vi "Parse Lights JSON.vi"(8 "error in":errorcluster, 10 "Light JSON":string="{\"1\":{\"name\": \"Hue Lamp\"},\"2\":{\"name\": \"Hue Lamp 1\"},\"3\":{\"name\": \"Hue Lamp 2\"}}") -> (0 "error out":errorcluster, 2 "Light Map":map{i32, T1}(c390))   [LabVIEW 2020, in "LMH-Hue.lvlib"]
uses:
  LMH-Hue.lvlib
  Type Defs/Light Data.ctl
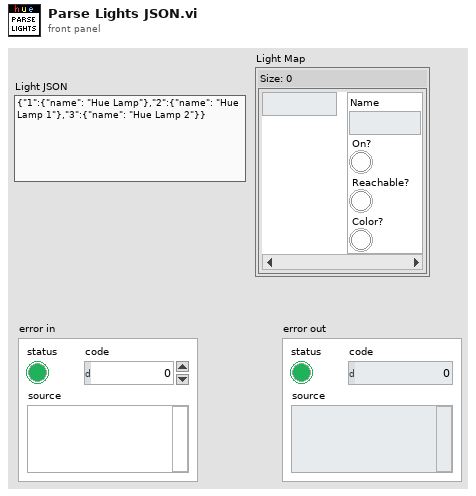
[diagram p1: front panel]
types:
  T1 = typedef "LMH-Hue.lvlib/Light Data.ctl" = cluster{"Name":string, "On?":bool, "Reachable?":bool, "Color?":bool}
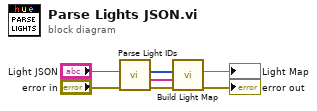
[diagram p0: block diagram]
diagram:
  n1 = call "Parse Light IDs.vi"("error in"="error in", "Light JSON"="Light JSON") -> ("error out"=w2:errorcluster, "Light Data"=w4:string[], "Light IDs"=w5:i32[])  [unwired: 7 in]
  n2 = call "Build Light Map.vi"("error in"=w2, "Light Data"=w4, "Light IDs"=w5) -> ("error out"=→"error out":errorcluster, "Light Map"=→"Light Map":map{i32, T1})  [unwired: 7 in]
